vi "series_front_coord.vi"(8 "error in (no error)":errorcluster, 10 "ROI Descriptor":T1 {"Contours"."Type" items=["No Selection", "Point", "Line", "Rectangle", "Oval", "Polygon", "Free", "Annulus", "Unused2", "Unused3", "Broken Line", "Free Hand Line", "Rotated Rectangle"]}, 11 "Image In":T3(plugin-control)) -> (0 "error out":errorcluster, 3 "Co ordinate System":T2)   [LabVIEW 2015]
uses:
  <vilib>/vision/Measure.llb/Edge Options.ctl
  <vilib>/vision/Measure.llb/Edge Polarity.ctl
  <vilib>/vision/Measure.llb/Straight Edge Options.ctl
  <vilib>/vision/Measure.llb/Straight Edge Process.ctl
  <vilib>/vision/NI_Vision_Development_Module.lvlib
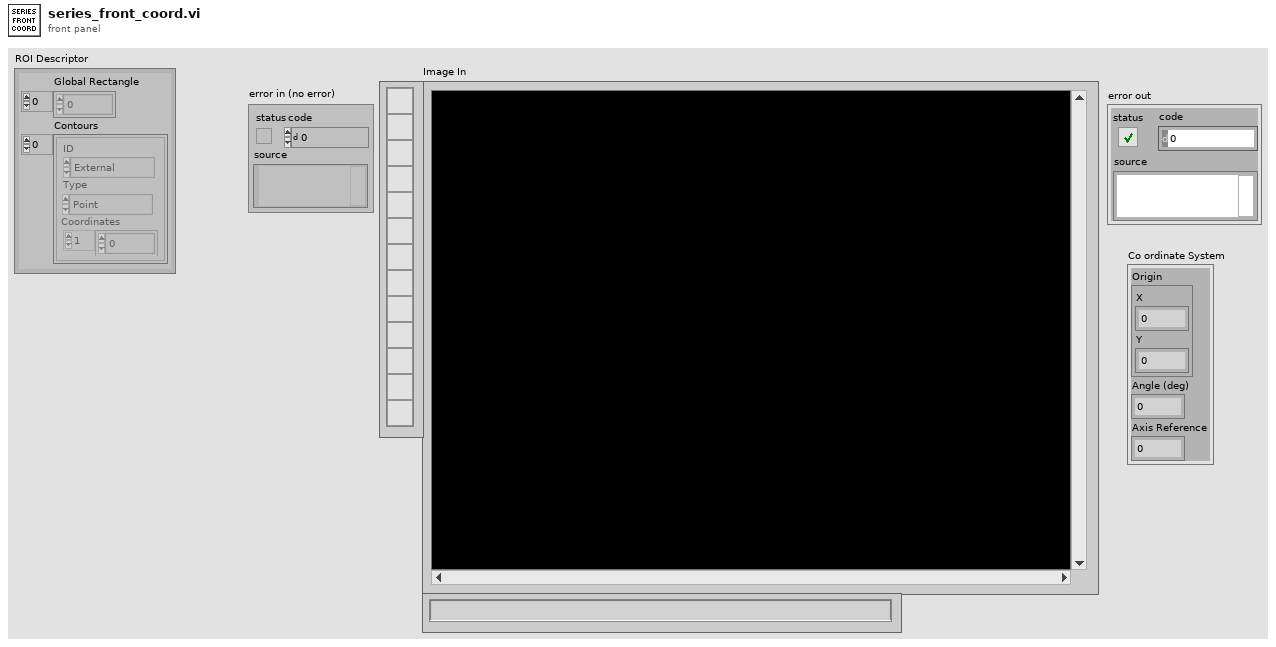
[diagram p1: front panel]
types:
  T1 = cluster{"Global Rectangle":i32[], "Contours":cluster{"ID":enum32{"External", "Internal"}, "Type":u32, "Coordinates":i32[]}[]}
  T2 = cluster{"Origin":cluster{"X":sgl, "Y":sgl}, "Angle (deg)":sgl, "Axis Reference":u32}
  T3 = typedef "IMAQ Image.ctl" = refnum<image>
  T4 = cluster{"Point 1":cluster{"X":sgl, "Y":sgl}, "Point 2":cluster{"X":sgl, "Y":sgl}}
  T5 = typedef "Straight Edge Options.ctl" = cluster{"Number of Lines":i32, "Type":T6, "Min. Score":dbl, "Max. Score":dbl, "Orientation":dbl, "Angle Range":dbl, "Angle Tolerance":dbl, "Step Size":u32, "Min. SNR (db)":dbl, "Min. Points (%)":dbl, "Hough Iterations":i32}
  T6 = typedef "Straight Edge Process.ctl" = enum32{"First Edge Rake", "Best Edge Rake", "Hough Edge Rake", "First Edge Projection", "Best Edge Projection"}
  T7 = typedef "Edge Options.ctl" = cluster{"Edge Polarity":T8, "Kernel Size":u32, "Width":u32, "Minimum Edge Strength":sgl, "Interpolation Type":enum32{"Zero Order", "Bilinear", "Quadratic", "Cubic", "Bilinear Fixed"}, "Data Processing Method":enum32{"Average", "Median"}}
  T8 = typedef "Edge Polarity.ctl" = u32
  T9 = cluster{"Point1 (Pixels)":cluster{"X":sgl, "Y":sgl}, "Point2 (Pixels)":cluster{"X":sgl, "Y":sgl}, "Point1 (Real-World)":cluster{"X":sgl, "Y":sgl}, "Point2 (Real-World)":cluster{"X":sgl, "Y":sgl}, "Angle (Pixel)":dbl, "Angle (Real-World)":dbl, "Score":dbl, "Straightness":dbl, "Average SNR (db)":dbl, "Calibration Valid":bool}[]
  T10 = cluster{"Point1 (Pixels)":cluster{"X":sgl, "Y":sgl}, "Point2 (Pixels)":cluster{"X":sgl, "Y":sgl}, "Point1 (Real-World)":cluster{"X":sgl, "Y":sgl}, "Point2 (Real-World)":cluster{"X":sgl, "Y":sgl}, "Angle (Pixel)":dbl, "Angle (Real-World)":dbl, "Score":dbl, "Straightness":dbl, "Average SNR (db)":dbl, "Calibration Valid":bool}
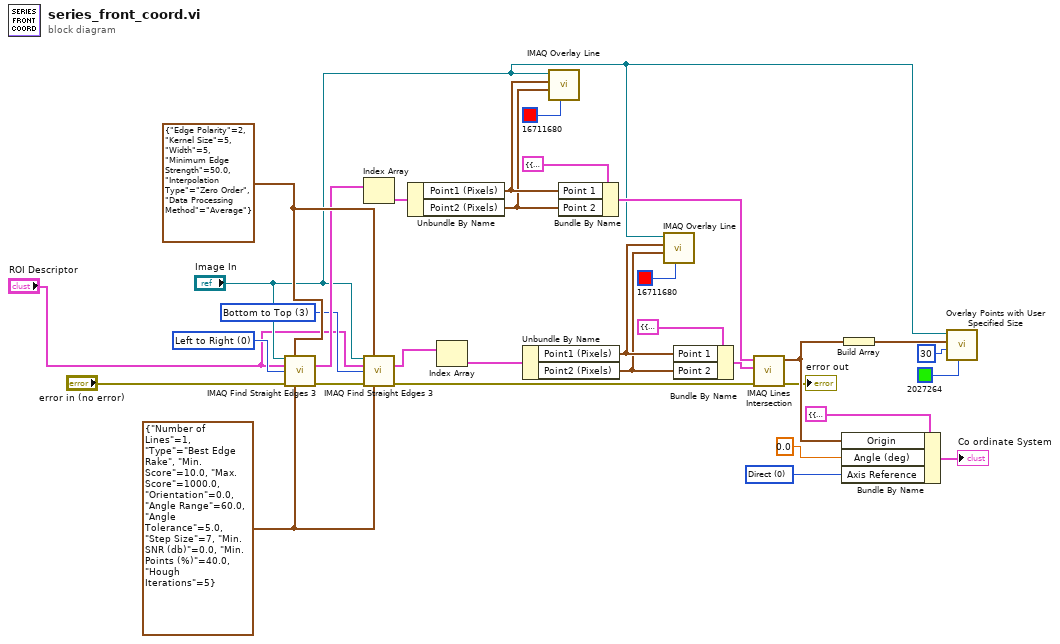
[diagram p0: block diagram]
diagram:
  w12 = u32 0 items=["Direct", "Indirect"] ("Axis Reference")
  w22 = u32 3 items=["Left to Right", "Right to Left", "Top to Bottom", "Bottom to Top"] ("Search Direction")
  w29 = T5 {"Number of Lines"=1, "Type"=enum."Best Edge Rake", "Min. Score"=10.0, "Max. Score"=1000.0, "Orientation"=0.0, "Angle Range"=60.0, "Angle Tolerance"=5.0, "Step Size"=7, "Min. SNR (db)"=0.0, "Min. Points (%)"=40.0, "Hough Iterations"=5} ("Line Options")
  w30 = T7 {"Edge Polarity"=2, "Kernel Size"=5, "Width"=5, "Minimum Edge Strength"=50.0, "Interpolation Type"=enum."Zero Order", "Data Processing Method"=enum."Average"} ("Edge Options")
  w32 = u32 0 items=["Left to Right", "Right to Left", "Top to Bottom", "Bottom to Top"] ("Search Direction")
  n1 = call "IMAQ Find Straight Edges 3"("Image"="Image In", "Edge Options"=w30, "ROI Descriptor"="ROI Descriptor", "Search Direction"=w32, "error in (no error)"="error in (no error)", "Line Options"=w29) -> ("Straight Edges"=w28:T9, "error out"=w31:errorcluster)  [unwired: 5 in, 3 out]
  n2 = Index Array(array=w28) -> (element=w26:T10)  [unwired: 1 in]
  n3 = call "IMAQ Find Straight Edges 3"("Image"="Image In", "Edge Options"=w30, "ROI Descriptor"="ROI Descriptor", "Search Direction"=w22, "error in (no error)"=w31, "Line Options"=w29) -> ("Straight Edges"=w27:T9, "error out"=w10:errorcluster)  [unwired: 5 in, 3 out]
  n4 = Unbundle By Name(w26) -> ("Point1 (Pixels)"=w17:cluster{"X":sgl, "Y":sgl}, "Point2 (Pixels)"=w16:cluster{"X":sgl, "Y":sgl})
  n5 = Index Array(array=w27) -> (element=w25:T10)  [unwired: 1 in]
  n6 = Unbundle By Name(w25) -> ("Point1 (Pixels)"=w15:cluster{"X":sgl, "Y":sgl}, "Point2 (Pixels)"=w14:cluster{"X":sgl, "Y":sgl})
  n7 = call "IMAQ Overlay Line"("Color"=u32 16711680, "End Point"=w16, "Start Point"=w17, "Image"="Image In") -> ()  [unwired: 6 in, 2 out]
  n8 = Bundle By Name(cluster=T4 {"Point 1"={"X"=0.0, "Y"=0.0}, "Point 2"={"X"=0.0, "Y"=0.0}} ("Line 1"), "Point 1"=w17, "Point 2"=w16) -> (w19:T4)
  n9 = call "IMAQ Overlay Line"("Color"=u32 16711680, "End Point"=w14, "Start Point"=w15, "Image"="Image In") -> ()  [unwired: 6 in, 2 out]
  n10 = Bundle By Name(cluster=T4 {"Point 1"={"X"=0.0, "Y"=0.0}, "Point 2"={"X"=0.0, "Y"=0.0}} ("Line 1"), "Point 1"=w15, "Point 2"=w14) -> (w18:T4)
  n11 = call "IMAQ Lines Intersection"("error in (no error)"=w10, "Line 2"=w18, "Line 1"=w19) -> ("error out"=→"error out":errorcluster, "Intersection Point"=w8:cluster{"X":sgl, "Y":sgl})  [unwired: 6 in, 1 out]
  n12 = Bundle By Name(cluster=T2 {"Origin"={"X"=0.0, "Y"=0.0}, "Angle (deg)"=0.0, "Axis Reference"=0} ("Coordinate System"), "Origin"=w8, "Angle (deg)"=sgl 0.0, "Axis Reference"=w12) -> (→"Co ordinate System":T2)
  n13 = Build Array(w8) -> (w7:cluster{"X":sgl, "Y":sgl}[])
  n14 = call "Overlay Points with User Specified Size.vi"("Color"=u32 2027264, "Point Diameter (5)"=u32 30, "Points"=w7, "Image In"="Image In") -> ()  [unwired: 6 in, 2 out]
